vi "loop-proj.vi"(11 "pixmap":u32[][](array[numeric])=array480x854[409920 elements] format="%.0x") -> (0 "Ymax":i32=406, 1 "Ymin":i32=100, 2 "Xmax":i32=740, 3 "Xmin":i32=127)   [LabVIEW 2025]
panel:
  in  "Rmin db":u8
  in  "Rmax db":u8=24
  in  "Gmin db":u8
  in  "Gmax db":u8=49
  in  "Bmin db":u8=100
  in  "Bmax db":u8=119
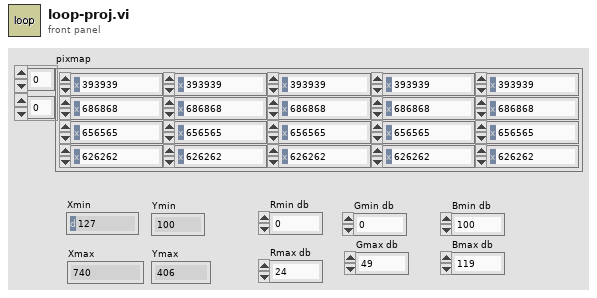
[diagram p1: front panel]
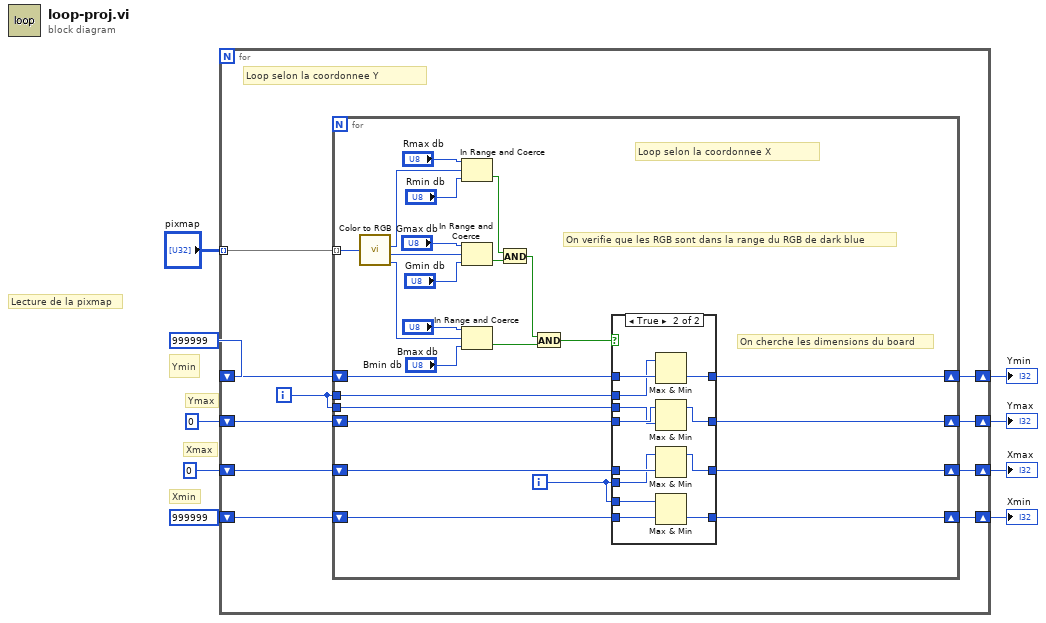
[diagram p0: block diagram]
diagram:
  # "Lecture de la pixmap"
  # "Ymax"
  # "Xmax"
  # "Ymin"
  # "Xmin"
  n1 = for {
    tunnel: "pixmap" -> [w10] mode=indexing
    shift-right: [w12] -> w3
    shift-left: 0 -> [w16]
    shift-right: [w13] -> w2
    shift-left: 999999 -> [w15]
    shift-right: [w19] -> w5
    shift-left: 999999 -> [w18]
    shift-right: [w14] -> w4
    shift-left: 0 -> [w17]
    i -> [w11]
    # "Loop selon la coordonnee Y"
    n2 = for {
      tunnel: w10 -> [w31] mode=indexing
      shift-right: [w30] -> w19
      shift-left: w18 -> [w27]
      shift-right: [w29] -> w14
      shift-left: w17 -> [w26]
      tunnel: w11 -> [w21]
      tunnel: w11 -> [w20]
      shift-right: [w22] -> w12
      shift-left: w16 -> [w25]
      shift-right: [w23] -> w13
      shift-left: w15 -> [w24]
      i -> [w28]
      # "Loop selon la coordonnee X"
      # "On cherche les dimensions du board"
      # "On verifie que les RGB sont dans la range du RGB de dark blue"
      n3 = call <vilib>:"Color to RGB.vi"("Color"=w31) -> ("R"=w45:u8, "G"=w44:u8, "B"=w37:u8)  [unwired: 1 out]
      n4 = In Range and Coerce(upper limit="Rmax db", x=w45, lower limit="Rmin db") -> (In Range?=w36:bool)  [unwired: 1 out]
      n5 = In Range and Coerce(upper limit="Gmax db", x=w44, lower limit="Gmin db") -> (In Range?=w35:bool)  [unwired: 1 out]
      n6 = In Range and Coerce(upper limit="Bmax db", x=w37, lower limit="Bmin db") -> (In Range?=w34:bool)  [unwired: 1 out]
      n7 = And(x=w36, y=w35) -> (x .and. y?=w33:bool)
      n8 = And(x=w33, y=w34) -> (x .and. y?=w32:bool)
      n9 = case shown="True" w32 {
        tunnel: w27 -> [w49 w59]
        tunnel: w28 -> [_ w61]
        tunnel: [w49 w60] -> w30
        tunnel: w26 -> [w48 w58]
        tunnel: [w48 w57] -> w29
        tunnel: w28 -> [_ w56]
        tunnel: w25 -> [w46 w55]
        tunnel: [w46 w54] -> w22
        tunnel: w24 -> [w47 w53]
        tunnel: [w47 w52] -> w23
        tunnel: w21 -> [_ w51]
        tunnel: w20 -> [_ w50]
        frame False {
        }
        frame True {
          n10 = Max & Min(x=w50, y=w53) -> (min(x,y)=w52:i32)  [unwired: 1 out]
          n11 = Max & Min(x=w55, y=w51) -> (max(x,y)=w54:i32)  [unwired: 1 out]
          n12 = Max & Min(x=w56, y=w58) -> (max(x,y)=w57:i32)  [unwired: 1 out]
          n13 = Max & Min(x=w61, y=w59) -> (min(x,y)=w60:i32)  [unwired: 1 out]
        }
      }
    }
  }
  "Xmin" <- w5
  "Ymin" <- w2
  "Xmax" <- w4
  "Ymax" <- w3
